vi "Keithley2400series_Meas.vi"(4 "MEAS:<f>":string, 5 "error in (no error)":errorcluster, 6 "MEAS mode, 0 Volt":u16, 7 "ОРЭ_th":dbl format="%.2f", 8 "VISA resource name in":refnum<visa-resource-name>) -> (0 "error out":errorcluster, 1 "SEE":bool, 2 "Замер":dbl format="%#.8g", 3 "VISA out":refnum<visa-resource-name>)   [LabVIEW 2014]
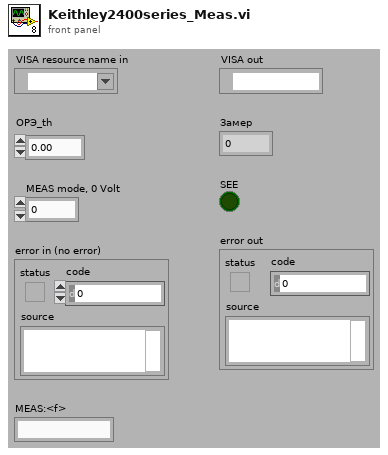
[diagram p1: front panel]
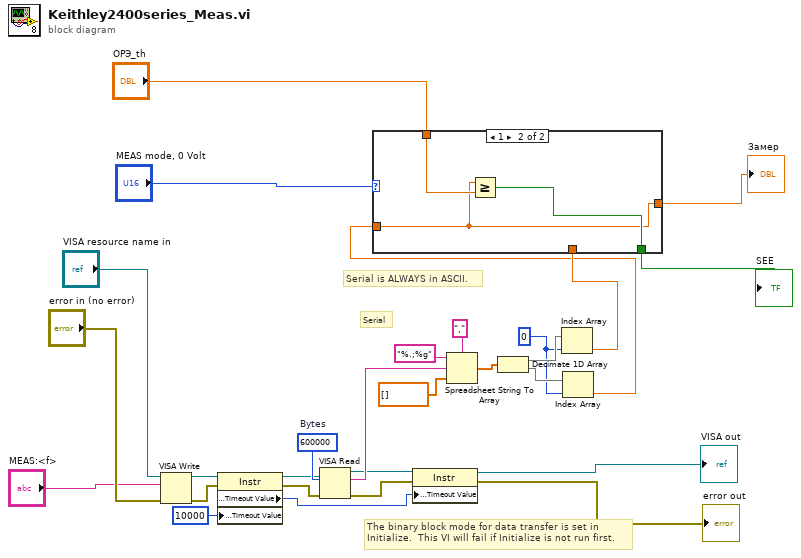
[diagram p0: block diagram]
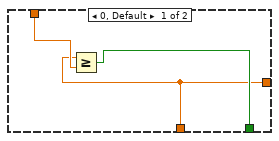
[diagram p2: hidden frame]
diagram:
  w12 = 0 ("index")
  w21 = u32 600000  # Bytes
  # "Serial is ALWAYS in ASCII."
  # "Serial"
  # "The binary block mode for data transfer is set in Initialize.  This VI will fail if Initialize is not run first."
  n1 = VISA Write(VISA resource name="VISA resource name in", write buffer="MEAS:<f>", error in (no error)="error in (no error)") -> (VISA resource name out=w22:refnum<visa-resource-name>, error out=w16:errorcluster)  [unwired: 1 out]
  n2 = property class="Instr"(reference=w22, error in=w16, "General Settings:Timeout Value"=u32 10000) -> (reference out=w17:refnum<visa-resource-name>, error out=w18:errorcluster, "General Settings:Timeout Value"=w27:u32)
  n3 = VISA Read(VISA resource name=w17, byte count=w21, error in (no error)=w18) -> (VISA resource name out=w19:refnum<visa-resource-name>, read buffer=w26:string, error out=w20:errorcluster)  [unwired: 1 out]
  n4 = property class="Instr"(reference=w19, error in=w20, "General Settings:Timeout Value"=w27) -> (reference out=→"VISA out":refnum<visa-resource-name>, error out=→"error out":errorcluster)
  n5 = Spreadsheet String To Array(delimiter (Tab)=",", format string="%.;%g", spreadsheet string=w26, array type (2D Dbl)=sgl[] []) -> (array=w15:sgl[])
  n6 = Decimate 1D Array(w15) -> (w14:sgl[], w13:sgl[])
  n7 = Index Array(array=w14, index=w12) -> (element=w11:sgl)
  n8 = Index Array(array=w13, index=w12) -> (element=w10:sgl)
  n9 = case shown="1" "MEAS mode, 0 Volt" {
    tunnel: w10 -> [_ w32]
    tunnel: w11 -> [w29 _]
    tunnel: "ОРЭ_th" -> [w31 w34]
    tunnel: [w30 w33] -> w28
    tunnel: [w29 w32] -> w2
    frame 0, Default {
      n10 = Greater Or Equal?(x=w29, y=w31) -> (x >= y?=w30:bool)
    }
    frame 1 {
      n11 = Greater Or Equal?(x=w32, y=w34) -> (x >= y?=w33:bool)
    }
  }
  "Замер" <- w2
  "SEE" <- w28
